vi "Main On Compile Action VI.vi"(8 "error in (no error)":errorcluster, 11 "Device Item Ref in":T1 format="%.0x") -> (0 "error out":errorcluster)   [LabVIEW 2020, in "RefMem DMA System Explorer.lvlib"]
uses:
  RefMem DMA System Explorer.lvlib
  <vilib>/NI VeriStand/Custom Device API/Custom Device Item Ref.ctl
  Shared/Compiled Settings Typedef.ctl
  Shared/Block descriptor.ctl
  Main On Compile Action VI_Parse DMA Block Prop.vi
  Shared/Constants.vi
  <vilib>/NI VeriStand/Custom Device API/NI VeriStand - Get Item Children.vi
  <vilib>/NI VeriStand/Custom Device API/NI VeriStand - Get Item GUID.vi
  <vilib>/NI VeriStand/Custom Device API/NI VeriStand - Get Item Property.vi
  <vilib>/NI VeriStand/Custom Device API/Get Item Property (U16).vi
  <vilib>/NI VeriStand/Custom Device API/Get Item Property (U32).vi
  Main On Compile Action VI_Get Buffer Index.vi
  <vilib>/NI VeriStand/Custom Device API/Set Item Property (Variant).vi
  <vilib>/NI VeriStand/Custom Device API/Custom Device API.lvlib
  Shared/RefMem DMA Shared.lvlib
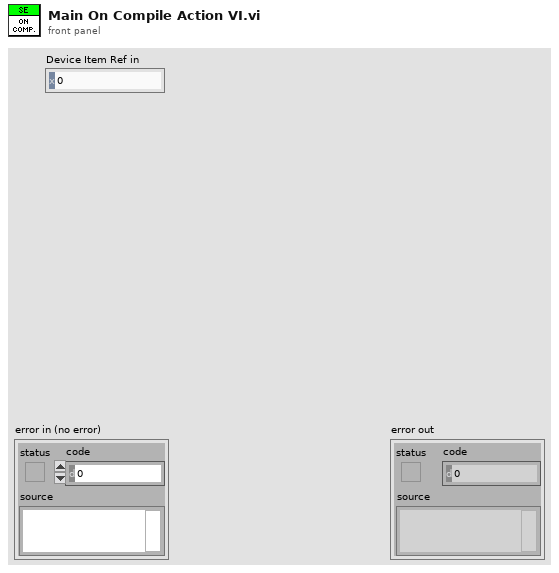
[diagram p1: front panel]
types:
  T1 = typedef "Custom Device API.lvlib/Custom Device Item Ref.ctl" = u64
  T2 = typedef "RefMem DMA Shared.lvlib/Compiled Settings Typedef.ctl" = cluster{"Read Block Descriptors":T3[], "max channel count bytes":u32, "Read":bool, "Write":bool, "Write Block Descriptors":T3[]}
  T3 = typedef "RefMem DMA Shared.lvlib/Block descriptor.ctl" = cluster{"Block Address in Bytes":u32, "Block Decimation \nchannel index":i32, "Transfer size":u32, "FIFO Indexes":i32[], "Channel index in block":i32[]}
  T4 = enum16{"open", "replace", "create", "open or create", "replace or create", "replace or create with confirmation"}
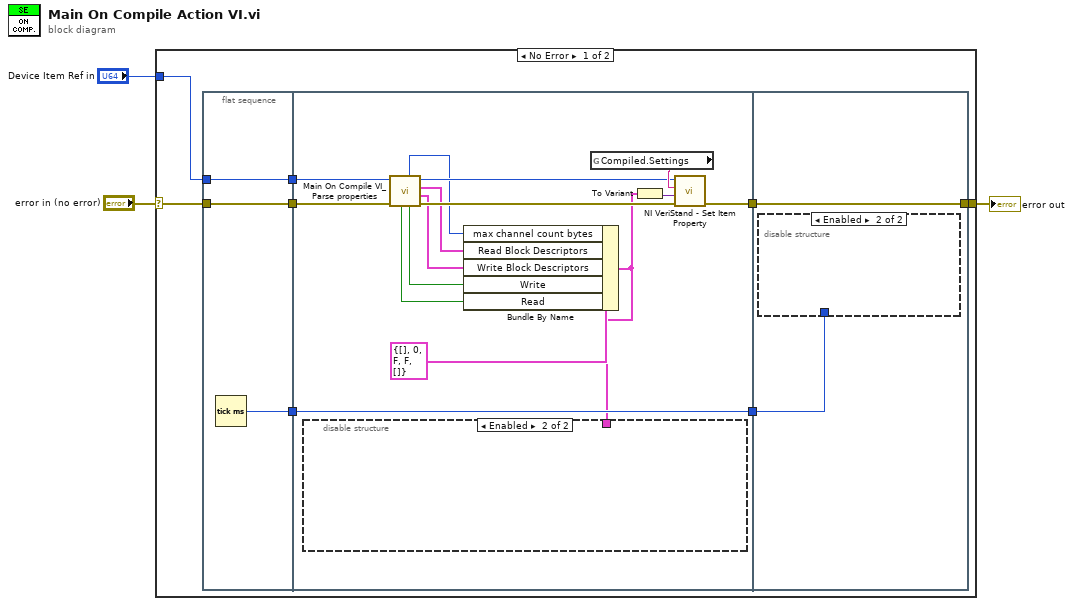
[diagram p0: block diagram]
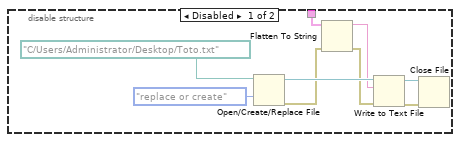
[diagram p2: hidden frame]
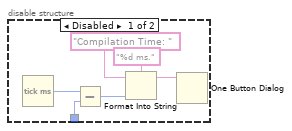
[diagram p3: hidden frame]
diagram:
  n1 = case shown="No Error" "error in (no error)" {
    selector: "error in (no error)" -> [w11 w47]
    tunnel: [w9 w47] -> w3
    tunnel: "Device Item Ref in" -> [w10 _]
    frame No Error {
      n2 = flat-sequence {
        tunnel: w11 -> [w13]
        tunnel: w10 -> [w14]
        tunnel: [w14] -> w8
        tunnel: [w13] -> w7
        tunnel: [w12] -> w6
        tunnel: w8 -> [w16]
        tunnel: w7 -> [w15]
        tunnel: w6 -> [w26]
        tunnel: [w29] -> w5
        tunnel: [w26] -> w4
        tunnel: [w40] -> w9
        tunnel: w5 -> [w40]
        tunnel: w4 -> [w39]
        frame #0 {
          n3 = Tick Count (ms)() -> (millisecond timer value=w12:u32)
        }
        frame #1 {
          n4 = call "Main On Compile VI_Parse properties.vi"("error in (no error)"=w15, "Device Reference"=w16) -> ("error out"=w27:errorcluster, "Write Block Descriptors"=w20:T3[], "Read Block Descriptors"=w21:T3[], "Device Ref out"=w25:T1, "Write"=w19:bool, "max channel count bytes"=w22:u32, "Read"=w18:bool)  [unwired: 3 in]
          n5 = Bundle By Name(cluster=T2 {"Read Block Descriptors"=[], "max channel count bytes"=0, "Read"=FALSE, "Write"=FALSE, "Write Block Descriptors"=[]} ("Compiled Settings"), "max channel count bytes"=w22, "Read Block Descriptors"=w21, "Write Block Descriptors"=w20, "Write"=w19, "Read"=w18) -> (w17:T2)
          n6 = disable-structure shown="Enabled" {
            disable-tunnel: w17 -> [w33 _]
            frame Disabled {
              n7 = Open/Create/Replace File(file path (use dialog)=path "C:/Users/Administrator/Desktop/Toto.txt", operation (0:open)=T4."replace or create") -> (refnum out=w38:refnum<file>, error out=w31:errorcluster)  [unwired: 4 in, 1 out]
              n8 = Flatten To String(anything=w33, error in (no error)=w31) -> (data string=w32:string, error out=w30:errorcluster)  [unwired: 2 in, 1 out]
              n9 = Write to Text File(file (use dialog)=w38, text=w32, error in=w30) -> (refnum out=w35:refnum<file>, error out=w34:errorcluster)  [unwired: 1 in, 1 out]
              n10 = Close File(refnum=w35, error in=w34) -> ()  [unwired: 2 out]
            }
            frame Enabled {
            }
          }
          n11 = global read "Constants.vi" "Compiled.Settings"() -> (w28:string)
          n12 = To Variant(anything=w17) -> (Variant=w24:variant)
          n13 = call-poly <vilib>:"NI VeriStand - Set Item Property.vi"("error in (no error)"=w27, "Value"=w24, "Property Name"=w28, "Item Ref in"=w25) -> ("error out"=w29:errorcluster)  [unwired: 5 in, 2 out]
        }
        frame #2 {
          n14 = disable-structure shown="Enabled" {
            disable-tunnel: w39 -> [w45 _]
            frame Disabled {
              n15 = Tick Count (ms)() -> (millisecond timer value=w46:u32)
              n16 = Subtract(x=w46, y=w45) -> (x-y=w44:u32)
              n17 = Format Into String(format string="%d ms.", initial string="Compilation Time: ", w44) -> (resulting string=w43:string)  [unwired: 1 in, 1 out]
              n18 = One Button Dialog(message=w43) -> ()  [unwired: 1 in, 1 out]
            }
            frame Enabled {
            }
          }
        }
      }
    }
    frame Error {
    }
  }
  "error out" <- w3
